vi "AlliGator Phasor Plot Image ROI Storage [MULT] v3.vi"(7 "Curent ROI Colors":u32[](array[colorbox]), 8 "Error In":errorcluster, 9 "Current ROI Descriptor(s)":T2[](array[typedef]) {"Contours"."Type" items=["No Selection", "Point", "Line", "Rectangle", "Oval", "Polygon", "Freehand Region", "Annulus", "Unused2", "Unused3", "Broken Line", "Freehand Line", "Rotated Rectangle"]}, 10 "Default Name(s) (\"ROI\")":string[](array[string]), 11 "Action":T1=enum."Update Current ROI Descriptor") -> (0 "Error Out":errorcluster, 1 "Current ROI Descriptors":T2[](array[typedef]) {"Contours"."Type" items=["No Selection", "Point", "Line", "Rectangle", "Oval", "Polygon", "Freehand Region", "Annulus", "Unused2", "Unused3", "Broken Line", "Freehand Line", "Rotated Rectangle"]}, 2 "Current ROI Names":string[](array[string]), 3 "Current Phasor Plot Image ROI":i32, 4 "Old ROI Name":string, 5 "Curent ROI Colors":u32[](array[colorbox]))   [LabVIEW 2021, in "AlliGator ROIs.lvlib"]
doc: "Handles multiple Phasor Plot image ROIs storage."
uses:
  AlliGator ROIs.lvlib
  AlliGator ROI Manager Actions.ctl
  Image/Named ROI Description.ctl
  AlliGator Variables List.ctl
  AlliGator Image ROI Event refnum.ctl
  Variant/Variant to Data/Variant to I32.vi
  <userlib>/_OpenG.lib/array/array.llb/Sort 1D Array (I32)__ogtk.vi
  Image/Image.lvlib
  AlliGator Globals, Variables & Constants.lvlib
  Variant/Variant to Data/Variant to Data.lvlib
  <userlib>/_OpenG.lib/array/array.llb/openg_array.lvlib
  Strings/Strings.lvlib
panel:
  # "see the AlliGator License on the block diagram (Ctrl+E or Window:Show Block Diagram)"
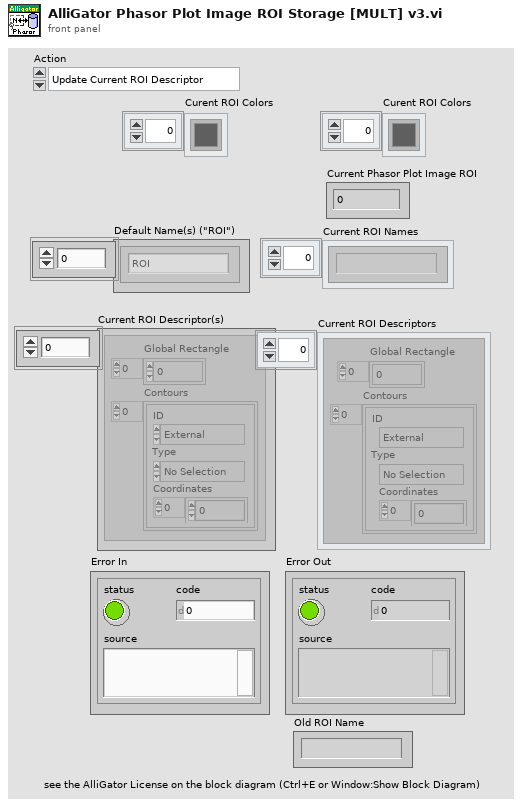
[diagram p1: front panel]
types:
  T1 = typedef "AlliGator ROIs.lvlib/AlliGator ROI Manager Actions.ctl" = enum16{"Undefined", "Delete Current ROI", "Delete All Unselected ROIs", "Delete Multiple ROIs", "Delete All ROIs", "Swap ROIs", "Insert ROI", "Update Current ROI Descriptor", "Rename Current ROI", "Store New ROI", "Store Multiple ROIs", "Select Next ROI", "Select Previous ROI", "Find Selected ROI", "Show All ROIs", "Update ROI Manager Window", "Merge All ROIs", "Unmerge ROI", "Set Selected ROI by ID"}
  T2 = typedef "ROI Descriptor" = cluster{"Global Rectangle":i32[], "Contours":cluster{"ID":enum32{"External", "Internal"}, "Type":u32, "Coordinates":i32[]}[]}
  T3 = typedef "AlliGator ROIs.lvlib/AlliGator Image ROI Event refnum.ctl" = refnum<user-event>
  T4 = typedef "AlliGator Globals, Variables & Constants.lvlib/AlliGator Variables List.ctl" = enum16{"---- GUI ----", "Initialization Status", "State Indicators Refnum", "Original AlliGator Menu Items", "Current Action Loop State", "Script in progress", "Playback", "Loop Playback", "Search ROI Used", "Search ROI", "Decay Graph Max Legend Size", "Intensity Graph Max Legend Size", "Decay Statistics Graph Max Legend Size", "Phasor Graph Max Legend Size", "Phasor Ratio Graph Max Legend Size", "Lifetime Graph Max Legend Size", "---- Files ----", "Export Dataset Frames as Individual Files", "Show Batch Export Help Balloons", "Frames in Dataset", "ptu File Frame Start Indices", "Current Frame in Dataset", "Current Frame Timestamp", "------ Python Plugins ------", "Python Plugins Information", "Python Session", "Valid Python Session?", "---- Source Image ----", "Dataset Loaded", "Dataset Metadata", "Dataset Channel", "Dataset Data Description", "Background Dataset Metadata", "Background Dataset Channel", "Background Dataset Data Description", "Background File Subtraction", "Background File Path", "Background File Pile-up Correction", "Background File Pixel Well Capacity", "Background File Scaling Factor", "Source Image ROIs", "Current Source Image ROI", "Source Image ROI Event Refnum", "X_Source Image Display Range", "X_Source Image Palette Information", "Source Image Palette List", "Source Image Scale", "Current Dataset Load Settings", "Source Image:ROI Overlay Color", "---- Image Profile Window ----", "Image Profile:Overlay ROI in Source Image", "Image Profile Window Event Refnum", "Image Profile:IntensityType", "Image Profile:Intensity Average Type", "Image Profile:Intensity-weighted SDV", "Image Profile:Box Profile Type", "Image Profile Window Open", "Image Profile:Plotted Fit Parameter", "X_Type of Displayed Image", "X_Time Gate Slider", "Dataset Path", "Source Image Overlay to Erase", "Is Displayed Image Accumulated", "White Light Image Modified", "Mask Image Modified", "Macrotime Gate Separation", "------ Phasor Graph -------", "Phasor Graph:Show Line", "---- Phasor Plot ---", "Phasor Plot Parameters Changed", "FLI Dataset Modified since last Phasor Plot Calculation", "Phasor Harmonics Data", "Selected Phasor Harmonics", "Phasor Harmonic Manager Event Refnum", "Phasor Plot ROIs", "Current Phasor Plot ROI", "Phasor Plot ROI Event Refnum", "Phasor Plot Image Reference Points", "Phasor Plot Computed", "Phasor Plot Palette Information", "Phasor Plot Palette List", "Phasor Ratio Palette Information", "Phasor Ratio Palette List", "Phasor Image Scale", "Phasor Plot Image Overlay to Erase", "Phasor Plot Image Elements to Update", "Current Phasor Plot Calculation Parameters", "Current Phasor Calibration Options", "Reset Cumulated Phasor Plot", "Phasor Ratio Reference 1", "Phasor Ratio Lifetime Reference 1", "Phasor Ratio Reference 1 Frequency", "Phasor Ratio Reference 2", "Phasor Ratio Lifetime Reference 2", "Phasor Ratio Reference 2 Frequency", "---- Decay Analysis ----", "Number of Selected Decays to Fit", "LS Fit Results", "LAR Fit Results", "BS Fit Results", "Last Decay Max - Min", "Best Fit Parameters", "Best Fit Parameter Names", "Actual Size X", "Actual Size Y", "Binning X", "Binning Y", "Actual # Gates", "Dataset Number", "Gates to...", "Gates Skipped", "Gates to keep", "Gate Step", "Gate Separation", "Reversed Gates", "Pile-up Correction", "Pixel Well Capacity", "Background Subtracted", "Background Subtraction Method", "Background Definition Range", "Background File (deprecated)", "Number of Dataset Accumulated", "Array of Accumulated Dataset Paths", "Do Averaged Datasets", "Destination File Path", "Process Plot Target", "Use 1/D as Phasor Frequency", "---- Decay Fit Parameter Map -----", "Decay Fit Parameter Map Palette Information", "Decay Fit Parameter Map Palette List", "Local Decay Graph Window Event Refnum", "------- Local Decay Window ---------", "Use normalized IRF for convolution", "----- Miscellaneous ----", "Skippable Dialog Windows Status"}
  T5 = typedef "Image.lvlib/Named ROI Description.ctl" = cluster{"ROI Descriptor":T2, "ROI Name":string, "Overlay Color":u32}
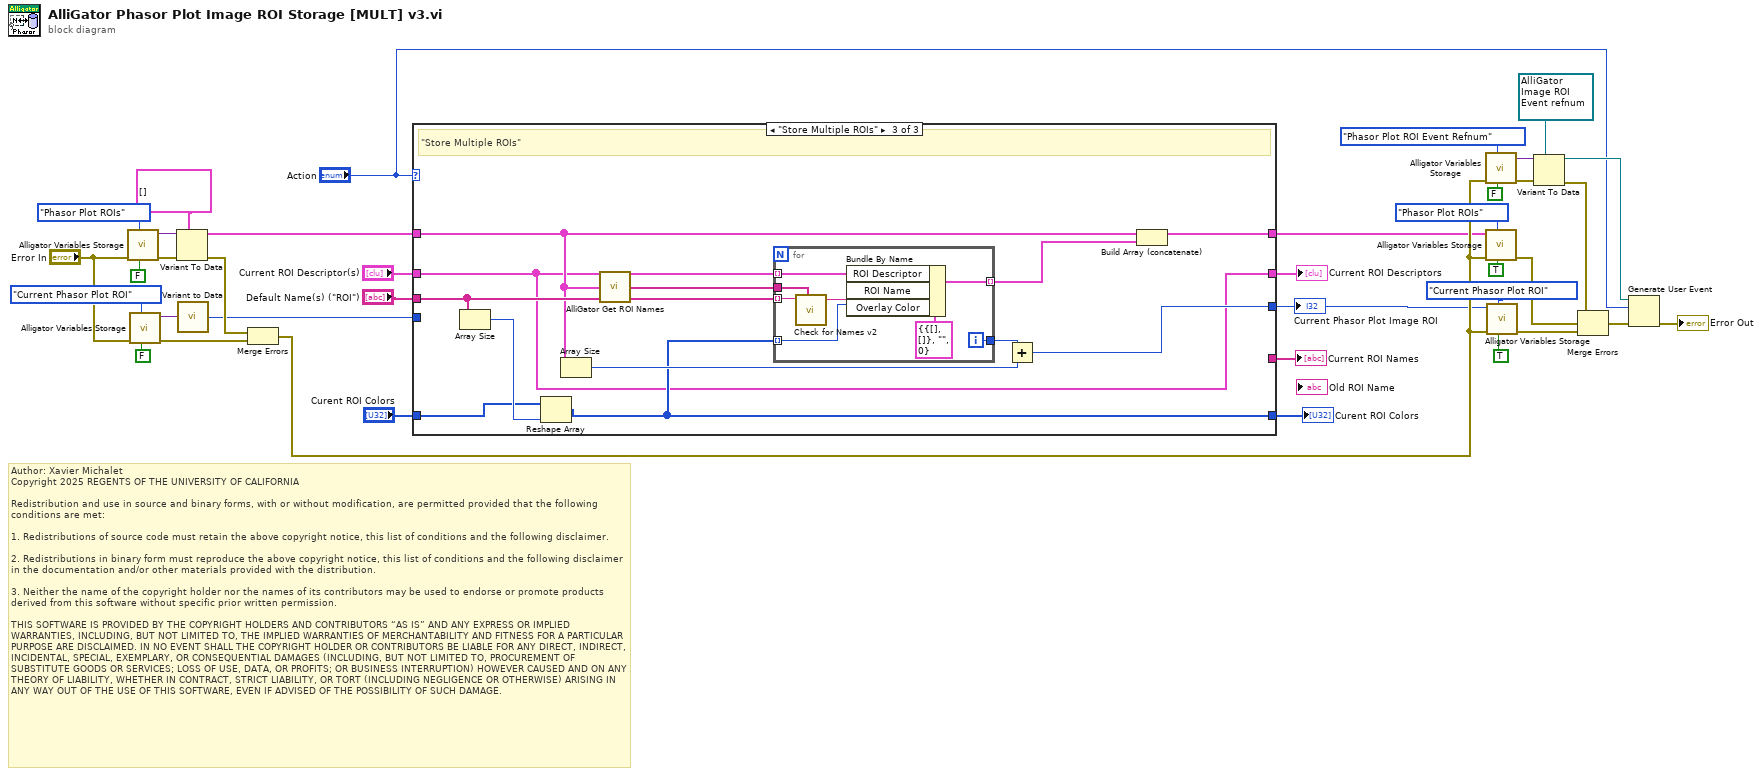
[diagram p0: block diagram]
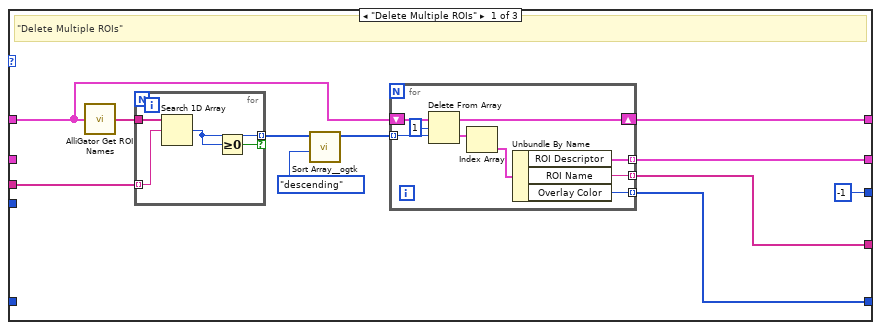
[diagram p2: hidden frame]
diagram:
  w14 = T3 refnum items=["Undefined", "Delete Current ROI", "Delete All Unselected ROIs", "Delete Multiple ROIs", "Delete All ROIs", "Swap ROIs", "Insert ROI", "Update Current ROI Descriptor", "Rename Current ROI", "Store New ROI", "Store Multiple ROIs", "Select Next ROI", "Select Previous ROI", "Find Selected ROI", "Show All ROIs", "Update ROI Manager Window", "Merge All ROIs", "Unmerge ROI", "Set Selected ROI by ID"] ("Source Image ROI Event Refnum")
  # "Author: Xavier Michalet\nCopyright 2025 REGENTS OF THE UNIVERSITY OF CALIFORNIA\n\nRedistribution and use in source and binary forms, with or without modification, are permitted provided that the following conditions are met:\n\n1. Redistributions of source code must retain the above copyright notice, this list of conditions and the following disclaimer.\n\n2. Redistributions in binary form must reproduce the above copyright notice, this list of conditions and the following disclaimer in the documentation and/or other materials provided with the distribution.\n\n3. Neither the name of the copyright holder nor the names of its contributors may be used to endorse or promote products derived from this software without specific prior written permission.\n\nTHIS SOFTWARE IS PROVIDED BY THE COPYRIGHT HOLDERS AND CONTRIBUTORS “AS IS” AND ANY EXPRESS OR IMPLIED WARRANTIES, INCLUDING, BUT NOT LIMITED TO, THE IMPLIED WARRANTIES OF MERCHANTABILITY AND FITNESS FOR A PARTICULAR PURPOSE ARE DISCLAIMED. IN NO EVENT SHALL THE COPYRIGHT HOLDER OR CONTRIBUTORS BE LIABLE FOR ANY DIRECT, INDIRECT, INCIDENTAL, SPECIAL, EXEMPLARY, OR CONSEQUENTIAL DAMAGES (INCLUDING, BUT NOT LIMITED TO, PROCUREMENT OF SUBSTITUTE GOODS OR SERVICES; LOSS OF USE, DATA, OR PROFITS; OR BUSINESS INTERRUPTION) HOWEVER CAUSED AND ON ANY THEORY OF LIABILITY, WHETHER IN CONTRACT, STRICT LIABILITY, OR TORT (INCLUDING NEGLIGENCE OR OTHERWISE) ARISING IN ANY WAY OUT OF THE USE OF THIS SOFTWARE, EVEN IF ADVISED OF THE POSSIBILITY OF SUCH DAMAGE."
  n1 = call "Alligator Variables Storage.vi"("Get(F)/Set"=FALSE, "AlliGator Variable"=AlliGator_Variables_List."Phasor Plot ROIs" ("Alligator Variable"), "Error In"="Error In") -> ("Error Out"=w36:errorcluster, "Data out"=w37:variant)  [unwired: 6 in, 1 out]
  n2 = call "Alligator Variables Storage.vi"("Get(F)/Set"=FALSE, "AlliGator Variable"=AlliGator_Variables_List."Current Phasor Plot ROI" ("Alligator Variable"), "Error In"="Error In") -> ("Error Out"=w26:errorcluster, "Data out"=w31:variant)  [unwired: 6 in, 1 out]
  n3 = Variant To Data(error in=w36, type=T5[] [] ("Stored ROIs in"), Variant=w37) -> (data=w11:T5[], error out=w25:errorcluster)
  n4 = call-poly "Variant to Data.vi"("Variant"=w31) -> ("Value"=w10:i32)  [unwired: 8 in]
  n5 = Merge Errors(w25, w26) -> (w17:errorcluster)
  n6 = case shown="\"Store Multiple ROIs\"" "Action" {
    tunnel: w11 -> [w43 w66 w72]
    tunnel: w10 -> [_ w64 _]
    tunnel: [w42 w66 w78] -> w7
    tunnel: [-1 ("Current ROI out") w64 w69] -> w6
    tunnel: "Current ROI Descriptor(s)" -> [_ w65 w67]
    tunnel: [w41 w65 w67] -> w5
    tunnel: "Default Name(s) (\"ROI\")" -> [w47 _ w75]
    tunnel: [w40 _ _] -> w4
    tunnel: [w39 w63 w68] -> w3
    tunnel: "Curent ROI Colors" -> [_ w63 w73]
    frame "Delete Multiple ROIs" {
      # "\"Delete Multiple ROIs\""
      n7 = call "AlliGator Get ROI Names.vi"("Stored ROIs in"=w43) -> ("ROI Name"=w48:string[])  [unwired: 8 in]
      n8 = for {
        tunnel: w48 -> [w62]
        tunnel: w47 -> [w61] mode=indexing
        tunnel: [w60] -> w46 mode=indexing if=w59
        n9 = Search 1D Array(1D array=w62, element=w61) -> (index of element=w60:i32)  [unwired: 1 in]
        n10 = Greater Or Equal To 0?(x=w60) -> (x >= 0?=w59:bool)
      }
      n11 = call-poly <userlib>:"Sort Array__ogtk.vi"("Order"=enum16{"ascending", "descending"}."descending", "Array in"=w46) -> ("Sorted Array out"=w44:i32[])  [unwired: 8 in, 1 out]
      n12 = for {
        tunnel: w44 -> [w58] mode=indexing
        shift-right: [w55] -> w42
        shift-left: w43 -> [w56]
        tunnel: [w52] -> w41 mode=indexing
        tunnel: [w51] -> w40 mode=indexing
        tunnel: [w50] -> w39 mode=indexing
        n13 = Delete From Array(array=w56, length=1, index=w58) -> (deleted portion=w54:T5[], array with subset deleted=w55:T5[])
        n14 = Index Array(array=w54) -> (element=w53:T5)  [unwired: 1 in]
        n15 = Unbundle By Name(w53) -> ("ROI Descriptor"=w52:T2, "ROI Name"=w51:string, "Overlay Color"=w50:u32)
      }
    }
    frame Default {
      # "Default"
    }
    frame "Store Multiple ROIs" {
      # "\"Store Multiple ROIs\""
      n16 = Array Size(array=w75) -> (size(s)=w74:i32)
      n17 = Reshape Array(w73, w74) -> (w68:u32[])
      n18 = Array Size(array=w72) -> (size(s)=w70:i32)
      n19 = call "AlliGator Get ROI Names.vi"("Stored ROIs in"=w72) -> ("ROI Name"=w76:string[])  [unwired: 8 in]
      n20 = for {
        tunnel: w67 -> [w84] mode=indexing
        tunnel: [w85] -> w77 mode=indexing
        tunnel: w75 -> [w82] mode=indexing
        tunnel: w76 -> [w83]
        tunnel: [w80] -> w71
        tunnel: w68 -> [w79] mode=indexing
        i -> [w80]
        n21 = call "Check for Names v2.vi"("New Name"=w82, "Name List"=w83) -> ("New Name"=w81:string)  [unwired: 4 in, 3 out]
        n22 = Bundle By Name(cluster=T5 {"ROI Descriptor"={"Global Rectangle"=[], "Contours"=[]}, "ROI Name"="", "Overlay Color"=0} ("Named ROI Description"), "ROI Descriptor"=w84, "ROI Name"=w81, "Overlay Color"=w79) -> (w85:T5)
      }
      n23 = Add(x=w71, y=w70) -> (x+y=w69:i32)
      n24 = Build Array (concatenate)(w72, w77) -> (w78:T5[])
    }
  }
  "Current ROI Descriptors" <- w5
  "Current Phasor Plot Image ROI" <- w6
  "Current ROI Names" <- w4
  "Curent ROI Colors" <- w3
  n25 = call "Alligator Variables Storage.vi"("Get(F)/Set"=FALSE, "AlliGator Variable"=AlliGator_Variables_List."Phasor Plot ROI Event Refnum" ("Alligator Variable"), "Error In"=w17) -> ("Error Out"=w16:errorcluster, "Data out"=w15:variant)  [unwired: 6 in, 1 out]
  n26 = call "Alligator Variables Storage.vi"("Get(F)/Set"=TRUE, "AlliGator Variable"=AlliGator_Variables_List."Phasor Plot ROIs" ("Alligator Variable"), "Error In"=w17, "Data in"=w7) -> ("Error Out"=w23:errorcluster)  [unwired: 5 in, 2 out]
  n27 = call "Alligator Variables Storage.vi"("Get(F)/Set"=TRUE, "AlliGator Variable"=AlliGator_Variables_List."Current Phasor Plot ROI" ("Alligator Variable"), "Error In"=w17, "Data in"=w6) -> ("Error Out"=w24:errorcluster)  [unwired: 5 in, 2 out]
  n28 = Variant To Data(error in=w16, type=w14, Variant=w15) -> (data=w13:T3, error out=w12:errorcluster)
  n29 = Merge Errors(w12, w23, w24) -> (w21:errorcluster)
  n30 = Generate User Event(user event=w13, event data cluster="Action", error in=w21) -> (error out=→"Error Out":errorcluster)  [unwired: 1 in, 1 out]
